vi "BLE - Get notifications.vi"(0 "COM Bluegiga in":refnum<visa-resource-name>, 3 "Error In":errorcluster) -> (7 "COM Bluegiga out":refnum<visa-resource-name>, 8 "Char handle":u16, 9 "Notified Data":u8[](array[numeric]), 10 "Error Out":errorcluster)   [LabVIEW 2016]
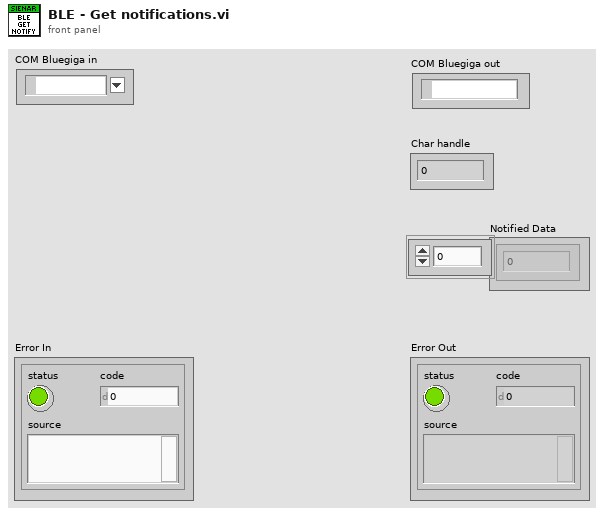
[diagram p1: front panel]
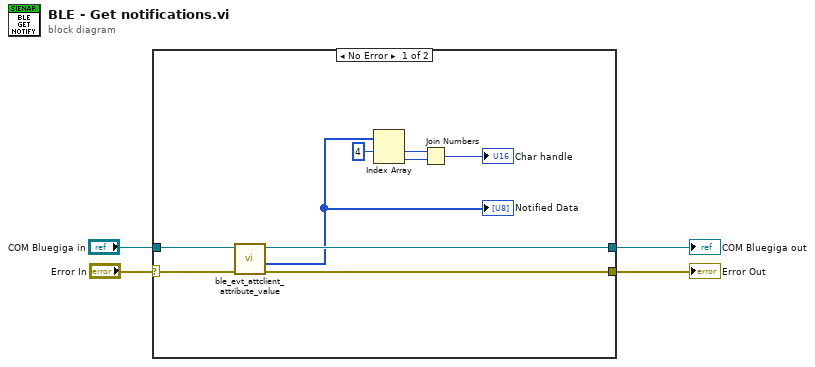
[diagram p0: block diagram]
diagram:
  n1 = case shown="No Error" "Error In" {
    selector: "Error In" -> [w13 w14]
    tunnel: [w12 w14] -> w3
    tunnel: "COM Bluegiga in" -> [w11 w15]
    tunnel: [w10 w15] -> w1
    frame No Error {
      n2 = call <vilib>:"ble_evt_attclient_attribute_value.vi"("error in (no error)"=w13, "COM Bluegiga in"=w11) -> ("error out"=w12:errorcluster, "full message package"=w9:u8[], "COM Bluegiga out"=w10:refnum<visa-resource-name>)  [unwired: 6 in, 1 out]
      "Notified Data" <- w9
      n3 = Index Array(array=w9, index #1=4 ("index")) -> (element #1=w6:u8, element #2=w7:u8)  [unwired: 1 in]
      n4 = Join Numbers(hi=w6, lo=w7) -> ((hi.lo)=→"Char handle":u16)
    }
    frame Error {
    }
  }
  "Error Out" <- w3
  "COM Bluegiga out" <- w1
